vi "Lead Screw Control.vi"(11 "Input Velocity":dbl) -> ()   [LabVIEW 2013]
panel:
  in  "Max":dbl=2.55
  in  "Min":dbl=0.15
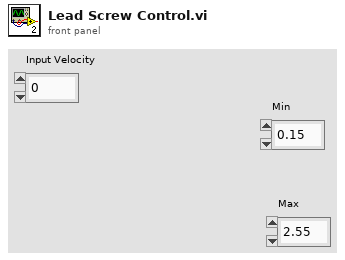
[diagram p1: front panel]
types:
  T1 = typedef "WPI_AnalogChannelDevRef.ctl" = cluster{"DevStatus":errorcluster, "Analog Module":T2, "Analog Channel":T3}
  T2 = typedef "FPGA_TypedefAnalogModule.ctl" = enum16{"Analog Module 1", "Analog Module 2"}
  T3 = typedef "FPGA_AIChannel.ctl" = enum8{"AI 1", "AI 2", "AI 3", "AI 4", "AI 5", "AI 6", "AI 7", "AI 8", "Invalid"}
  T4 = typedef "WPI_DigitalInputDevRef.ctl" = cluster{"DevStatus":errorcluster, "DIO Channel":T5, "Digital Module":T6}
  T5 = typedef "FPGA_DIOChannel.ctl" = enum8{"DIO 1", "DIO 2", "DIO 3", "DIO 4", "DIO 5", "DIO 6", "DIO 7", "DIO 8", "DIO 9", "DIO 10", "DIO 11", "DIO 12", "DIO 13", "DIO 14", "Invalid"}
  T6 = typedef "FPGA_TypedefDigitalModule.ctl" = enum16{"Digital Module 1", "Digital Module 2"}
  T7 = typedef "WPI_MotorControlDeviceRef.ctl" = cluster{"DeviceStatus":errorcluster, "Type":enum16{"PWM", "CAN"}, "PWM":cluster{"Digital Module":T6, "PWM Channel":T8, "DeadBand":T9}, "CAN":cluster{"Device Number":u8, "Control Mode":T10, "Semaphore":T11, "Max Vout":dbl}, "Invert":bool, "TransformRef":T12, "InvTransformRef":T12}
  T8 = typedef "FPGA_DIOPWMChannel.ctl" = enum8{"PWM 1", "PWM 2", "PWM 3", "PWM 4", "PWM 5", "PWM 6", "PWM 7", "PWM 8", "PWM 9", "PWM 10", "Invalid"}
  T9 = typedef "WPI_PWMDeadband.ctl" = cluster{"Name":string, "maxPositivePwm":i32, "minPositivePwm":i32, "centerPwm":i32, "maxNegativePwm":i32, "minNegativePwm":i32, "angularRange":u16}
  T10 = typedef "WPI_CANJaguar_ControlMode.ctl" = enum8{"Percent VBus", "Current", "Speed", "Position", "Voltage"}
  T11 = typedef "Semaphore RefNum" = refnum<k1>
  T12 = typedef "WPI_PWMTransform_ConPane.ctl" = refnum<vi>
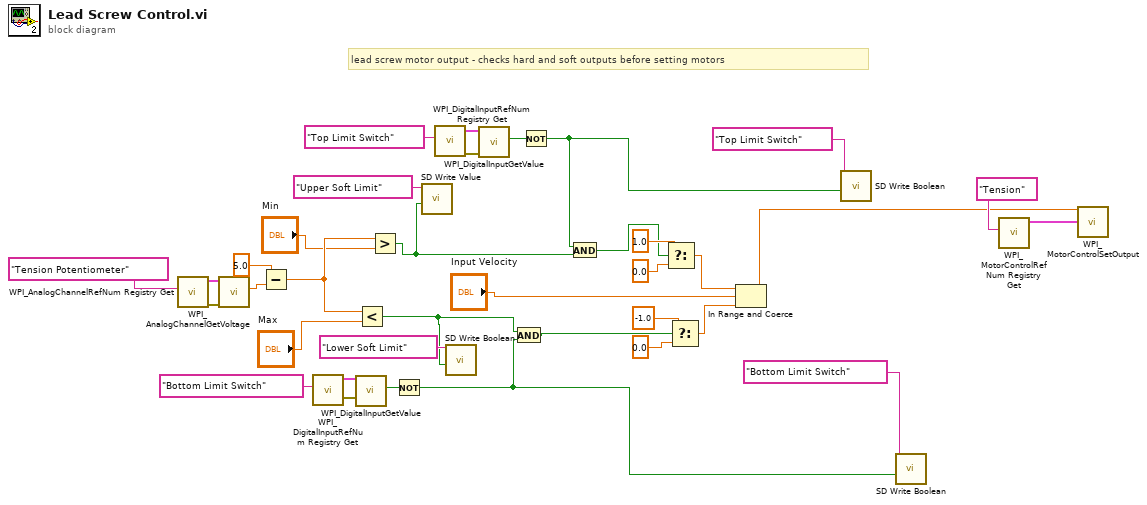
[diagram p0: block diagram]
diagram:
  # "lead screw motor output - checks hard and soft outputs before setting motors"
  n1 = call <vilib>:"WPI_AnalogChannelRefNum Registry Get.vi"("refnum name"="Tension Potentiometer") -> ("error out"=w18:errorcluster, "AIDeviceRef"=w17:T1)  [unwired: 9 in]
  n2 = call <vilib>:"WPI_AnalogChannelGetVoltage.vi"("error in (no error)"=w18, "AIDeviceRef"=w17) -> ("Voltage"=w15:dbl)  [unwired: 7 in, 2 out]
  n3 = Subtract(x=5.0, y=w15) -> (x-y=w12:dbl)
  n4 = call <vilib>:"WPI_DigitalInputRefNum Registry Get.vi"("refnum name"="Bottom Limit Switch") -> ("error out"=w32:errorcluster, "DigitalInputDevRef"=w34:T4)  [unwired: 9 in]
  n5 = call <vilib>:"WPI_DigitalInputGetValue.vi"("error in (no error)"=w32, "DigitalInputDevRef"=w34) -> ("Value"=w19:bool)  [unwired: 7 in, 2 out]
  n6 = Less?(x=w12, y="Max") -> (x < y?=w1:bool)
  n7 = Greater?(x=w12, y="Min") -> (0:w5:bool)
  n8 = Not(x=w19) -> (.not. x?=w10:bool)
  n9 = call-poly <vilib>:"SD Write Value.vi"("Boolean"=w5, "Name"="Upper Soft Limit") -> ()  [unwired: 8 in, 2 out]
  n10 = call <vilib>:"WPI_DigitalInputRefNum Registry Get.vi"("refnum name"="Top Limit Switch") -> ("error out"=w31:errorcluster, "DigitalInputDevRef"=w36:T4)  [unwired: 9 in]
  n11 = call <vilib>:"SD Write Boolean.vi"("Boolean"=w1, "Name"="Lower Soft Limit") -> ()  [unwired: 8 in, 2 out]
  n12 = call <vilib>:"WPI_DigitalInputGetValue.vi"("error in (no error)"=w31, "DigitalInputDevRef"=w36) -> ("Value"=w20:bool)  [unwired: 7 in, 2 out]
  n13 = And(x=w1, y=w10) -> (x .and. y?=w11:bool)
  n14 = Not(x=w20) -> (.not. x?=w13:bool)
  n15 = And(x=w13, y=w5) -> (x .and. y?=w9:bool)
  n16 = Select(t=1.0, s=w9, f=0.0) -> (s? t:f=w23:dbl)
  n17 = Select(t=-1.0, s=w11, f=0.0) -> (s? t:f=w24:dbl)
  n18 = In Range and Coerce(upper limit=w23, x="Input Velocity", lower limit=w24) -> (coerced(x)=w8:dbl)  [unwired: 1 out]
  n19 = call <vilib>:"SD Write Boolean.vi"("Boolean"=w13, "Name"="Top Limit Switch") -> ()  [unwired: 8 in, 2 out]
  n20 = call <vilib>:"SD Write Boolean.vi"("Boolean"=w10, "Name"="Bottom Limit Switch") -> ()  [unwired: 8 in, 2 out]
  n21 = call <vilib>:"WPI_MotorControlRefNum Registry Get.vi"("refnum name"="Tension") -> ("MotorControlDevRef"=w30:T7)  [unwired: 9 in, 1 out]
  n22 = call <vilib>:"WPI_MotorControlSetOutput.vi"("Output"=w8, "MotorControlDevRef"=w30) -> ()  [unwired: 7 in, 3 out]
